vi "DE_map.vi"(10 "din":cdb[](array[numeric])) -> (2 "out_bits":u8[](array[numeric]))   [LabVIEW 2010]
uses:
  <vilib>/addons/Modulation/niDMT.lvlib
  <vilib>/addons/Modulation/Digital/General/MT Generate Bits (Galois, PN Order).vi
  <vilib>/addons/Modulation/Digital/Support/Controls/Pack Bits Parameters.ctl
panel:
  out "x = y?":bool[](array[boolean])
  out "大小 2":i32
  out "output integers":i32[](array[numeric])
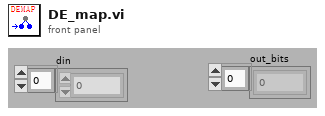
[diagram p1: front panel]
types:
  T1 = typedef "niDMT.lvlib/Pack Bits Parameters.ctl" = enum16{"Unsigned", "Signed"}
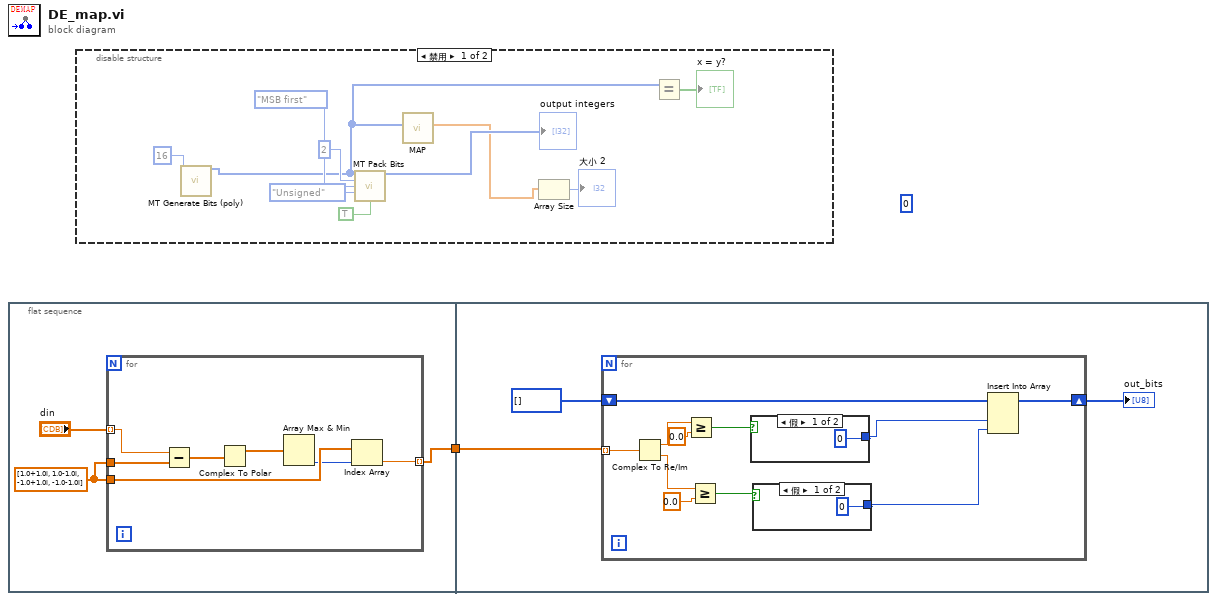
[diagram p0: block diagram]
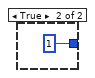
[diagram p2: hidden frame]
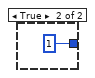
[diagram p3: hidden frame]
diagram:
  (unwired) u8 0
  n1 = flat-sequence {
    tunnel: [w2] -> w1
    tunnel: w1 -> [w12]
    frame #0 {
      w4 = cdb[] [1.0+1.0i, 1.0-1.0i, -1.0+1.0i, -1.0-1.0i]
      n2 = for {
        tunnel: w4 -> [w11]
        tunnel: w4 -> [w8]
        tunnel: [w6] -> w2 mode=indexing
        tunnel: "din" -> [w5] mode=indexing
        n3 = Subtract(x=w5, y=w11) -> (x-y=w10:cdb[])
        n4 = Complex To Polar(r * e^(i*theta)=w10) -> (r=w9:dbl[])  [unwired: 1 out]
        n5 = Array Max & Min(array=w9) -> (min index (indices)=w7:i32)  [unwired: 3 out]
        n6 = Index Array(array=w8, index=w7) -> (element=w6:cdb)
      }
    }
    frame #1 {
      n7 = for {
        tunnel: w12 -> [w25] mode=indexing
        shift-right: [w15] -> w13
        shift-left: u8[] [] -> [w18]
        n8 = Complex To Re/Im(x + iy=w25) -> (x=w24:dbl, y=w19:dbl)
        n9 = Greater Or Equal?(x=w24, y=0.0) -> (x >= y?=w22:bool)
        n10 = Greater Or Equal?(x=w19, y=0.0) -> (x >= y?=w20:bool)
        n11 = case shown="假" w22 {
          tunnel: [u8 0 u8 1] -> w17
          frame False {
          }
          frame True {
          }
        }
        n12 = case shown="假" w20 {
          tunnel: [u8 0 u8 1] -> w16
          frame False {
          }
          frame True {
          }
        }
        n13 = Insert Into Array(array=w18, new element #1=w17, new element #2=w16) -> (w15:u8[])  [unwired: 1 in]
      }
      "out_bits" <- w13
    }
  }
  n14 = disable-structure shown="禁用" {
    frame Disabled {
      n15 = call-poly <vilib>:"MT Generate Bits (poly).vi"("total bits (128)"=16) -> ("output bit stream"=w32:i8[])  [unwired: 12 in, 2 out]
      n16 = call <vilib>:"MT Pack Bits.vi"("input bit stream"=w32, "bits per integer"=2, "packed bit order"=enum16{"MSB first", "LSB first"}."MSB first", "integer format"=Pack_Bits_Parameters."Unsigned", "reset ? (T)"=TRUE) -> ("output integers"=→"output integers":i32[])  [unwired: 9 in, 1 out]
      n17 = call "MAP.vi"("input bit stream"=w32) -> ("dout"=w30:cdb[])  [unwired: 10 in]
      n18 = Array Size(array=w30) -> (size(s)=→"大小 2":i32)
      n19 = Equal?(x=w32) -> (x = y?=→"x = y?":bool[])  [unwired: 1 in]
    }
    frame Enabled {
    }
  }
